vi "check log file info default values.vi"(10 "Target Type":T1, 11 "log file info in":T2={"Log Directory"="/c/ni-rt/NIVeriStand/Logs", "Base Name"="AIM664log", "Timestamp"=FALSE, "Enabled"=FALSE}) -> (3 "log file info out":T2={"Log Directory"="/c/ni-rt/NIVeriStand/Logs", "Base Name"="AIM664log", "Timestamp"=FALSE, "Enabled"=FALSE})   [LabVIEW 2020]
uses:
  logFileInfo_types.ctl
  <vilib>/NI VeriStand/Custom Device API/Custom Device Target Type.ctl
  <vilib>/NI VeriStand/Custom Device API/Custom Device API.lvlib
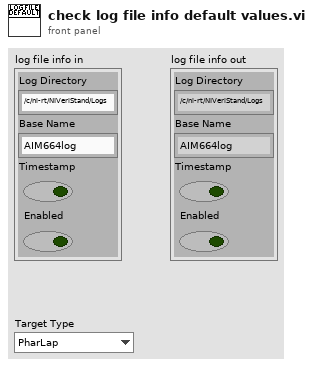
[diagram p1: front panel]
types:
  T1 = typedef "Custom Device API.lvlib/Custom Device Target Type.ctl" = enum16{"PharLap", "VxWorks", "Windows", "Linux_32_ARM", "Linux_x64"}
  T2 = typedef "logFileInfo_types.ctl" = cluster{"Log Directory":string, "Base Name":string, "Timestamp":bool, "Enabled":bool}
  T3 = cluster{"Log Directory":string, "Base Name":string, "Log Timestamp":bool}
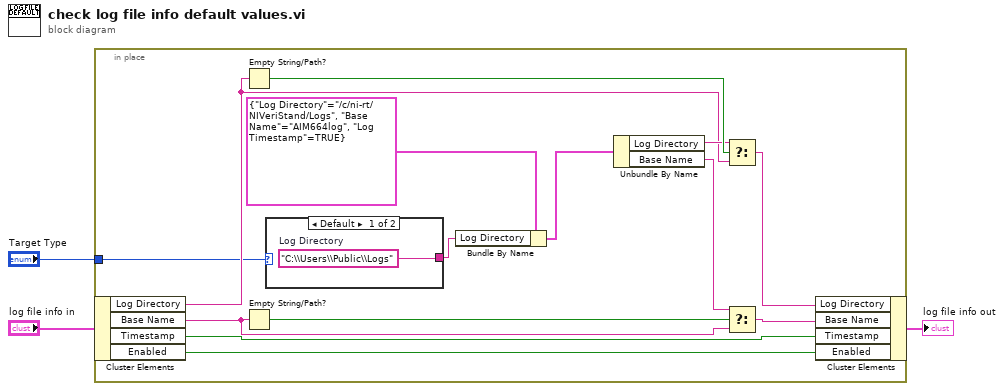
[diagram p0: block diagram]
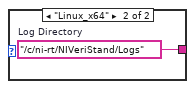
[diagram p2: hidden frame]
diagram:
  n1 = in-place {
    in-place-border: "Target Type" -> [w5]
    n2 = in-place-cluster #1("log file info in") -> ("Log Directory"=w14:string, "Base Name"=w11:string, "Timestamp"=w9:bool, "Enabled"=w8:bool)
    n3 = Empty String/Path?(string/path=w14) -> (empty?=w17:bool)
    n4 = Empty String/Path?(string/path=w11) -> (empty?=w16:bool)
    n5 = case shown="Default" w5 {
      tunnel: [w18 w19] -> w4
      frame Default {
        w18 = "C:\\Users\\Public\\Logs"  # Log Directory
      }
      frame "Linux_x64" {
        w19 = "/c/ni-rt/NIVeriStand/Logs"  # Log Directory
      }
    }
    n6 = Bundle By Name(cluster=T3 {"Log Directory"="/c/ni-rt/NIVeriStand/Logs", "Base Name"="AIM664log", "Log Timestamp"=TRUE} ("log file info"), "Log Directory"=w4) -> (w6:T3)
    n7 = Unbundle By Name(w6) -> ("Log Directory"=w15:string, "Base Name"=w12:string)
    n8 = Select(t=w15, s=w17, f=w14) -> (s? t:f=w13:string)
    n9 = Select(t=w12, s=w16, f=w11) -> (s? t:f=w10:string)
    n10 = in-place-cluster #1("Log Directory"=w13, "Base Name"=w10, "Timestamp"=w9, "Enabled"=w8) -> (→"log file info out":T2)
  }
